vi "Run Process.vi"(8 "error in (no error)":errorcluster, 11 "ChartProc in":refnum<class "ChartProc.lvclass">) -> (0 "error out":errorcluster, 3 "ChartProc out":refnum<class "ChartProc.lvclass">)   [LabVIEW 2020, in "LAF2024Q2.lvlib" / "ChartProc.lvclass"]
uses:
  ChartProc.lvclass
  C:/dev/lv 2020/laf-2024-q2/LAF2024Q2/CoolAppProcess/CoolAppProcess.lvclass
  ChartProc.lvclass/ChartProc.ctl
  CoolAppProcess/CoolAppProcess.lvclass
panel:
  out "Chart":dbl(graph)
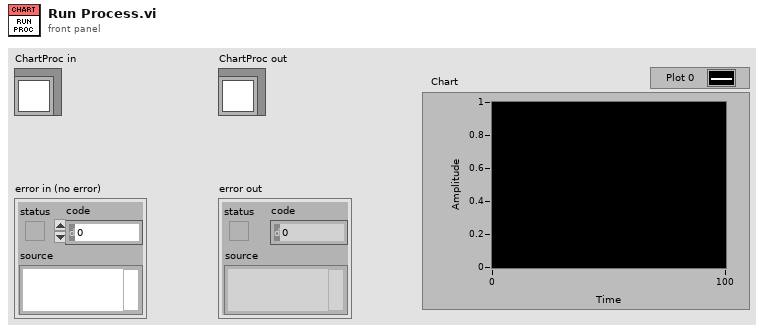
[diagram p1: front panel]
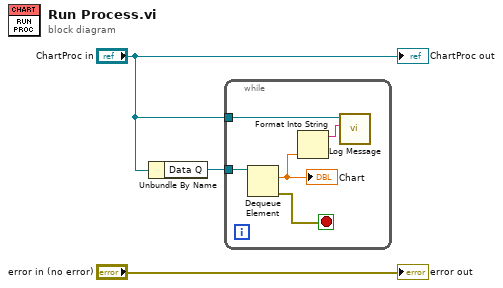
[diagram p0: block diagram]
diagram:
  n1 = Unbundle By Name("ChartProc in") -> ("Data Q"=w2:refnum<queue>)
  n2 = while {
    tunnel: w2 -> [w8]
    tunnel: "ChartProc in" -> [w6]
    stop <- w7 stop-if-true
    n3 = Dequeue Element(queue=w8) -> (element=w5:dbl, error out=w7:errorcluster)  [unwired: 2 in, 2 out]
    "Chart" <- w5
    n4 = Format Into String(w5) -> (resulting string=w4:string)  [unwired: 3 in, 1 out]
    n5 = call "Log Message.vi"("Message"=w4, "CoolAppProcess in"=w6) -> ()  [unwired: 8 in, 2 out]
  }
  "error out" <- "error in (no error)"
  "ChartProc out" <- "ChartProc in"
